vi "IP Address.vi"(11 "Data":u8[](array[numeric])) -> (3 "IP Address":string)   [LabVIEW 2017]
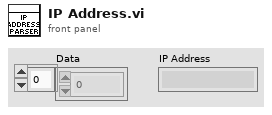
[diagram p1: front panel]
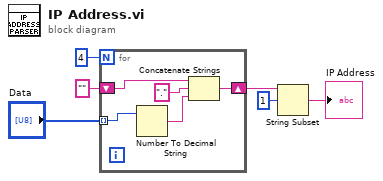
[diagram p0: block diagram]
diagram:
  n1 = for {
    N: 4 -> [_]
    shift-right: [w11] -> w3
    shift-left: "" -> [w10]
    tunnel: "Data" -> [w7] mode=indexing
    n2 = Number To Decimal String(number=w7) -> (decimal integer string=w9:string)  [unwired: 1 in]
    n3 = Concatenate Strings(w10, "." ("string"), w9) -> (w11:string)
  }
  n4 = String Subset(string=w3, offset (0)=1) -> (substring=→"IP Address":string)  [unwired: 1 in]
